vi "HCSD_125_scan.vi"() -> ()   [LabVIEW 2013]
uses:
  <vilib>/Utility/file.llb/Write To Spreadsheet File (string).vi
  <userlib>/caLab/Private/Get_PV-1D.vi
panel:
  in  "Diff SD":dbl=0.05
  out "refresh_ms":u32=51
  out "refresh (ms)":u32(graph)=51
  in  "diff HC":dbl=0.02 format="%#_13f"
  in  "stop":bool
  in  "Check period (ms)":u32=50 max=10
  out "Diff list":string[][](array[string])
  out "check loop":i32=1821
  out "EVENTs":i32
  out "Program Start Time":dbl=3594202634.3800077
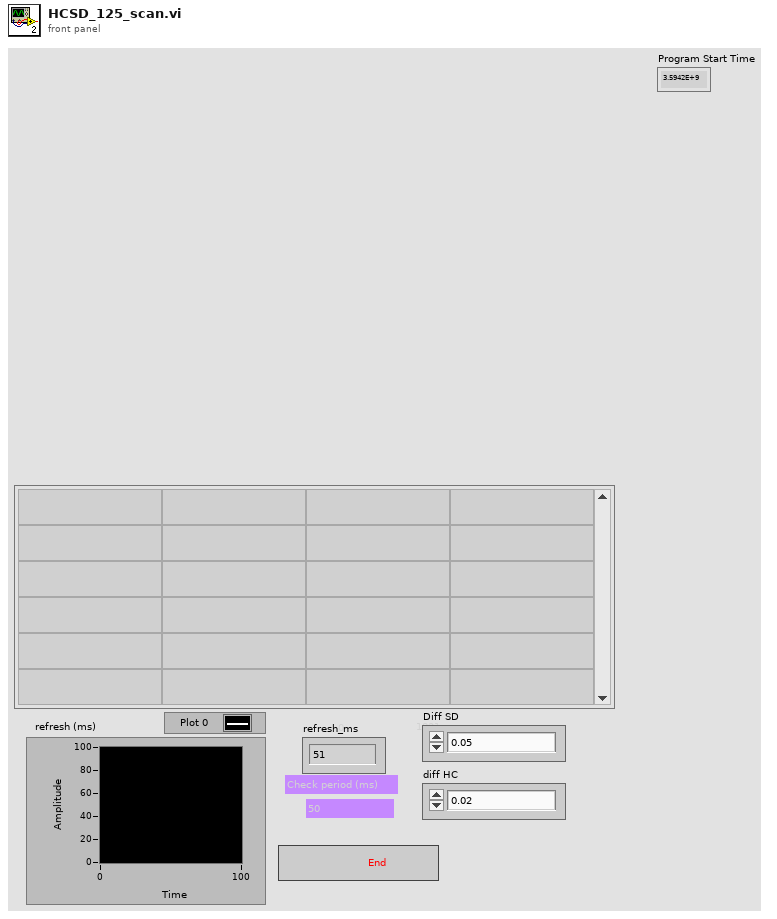
[diagram p1: front panel]
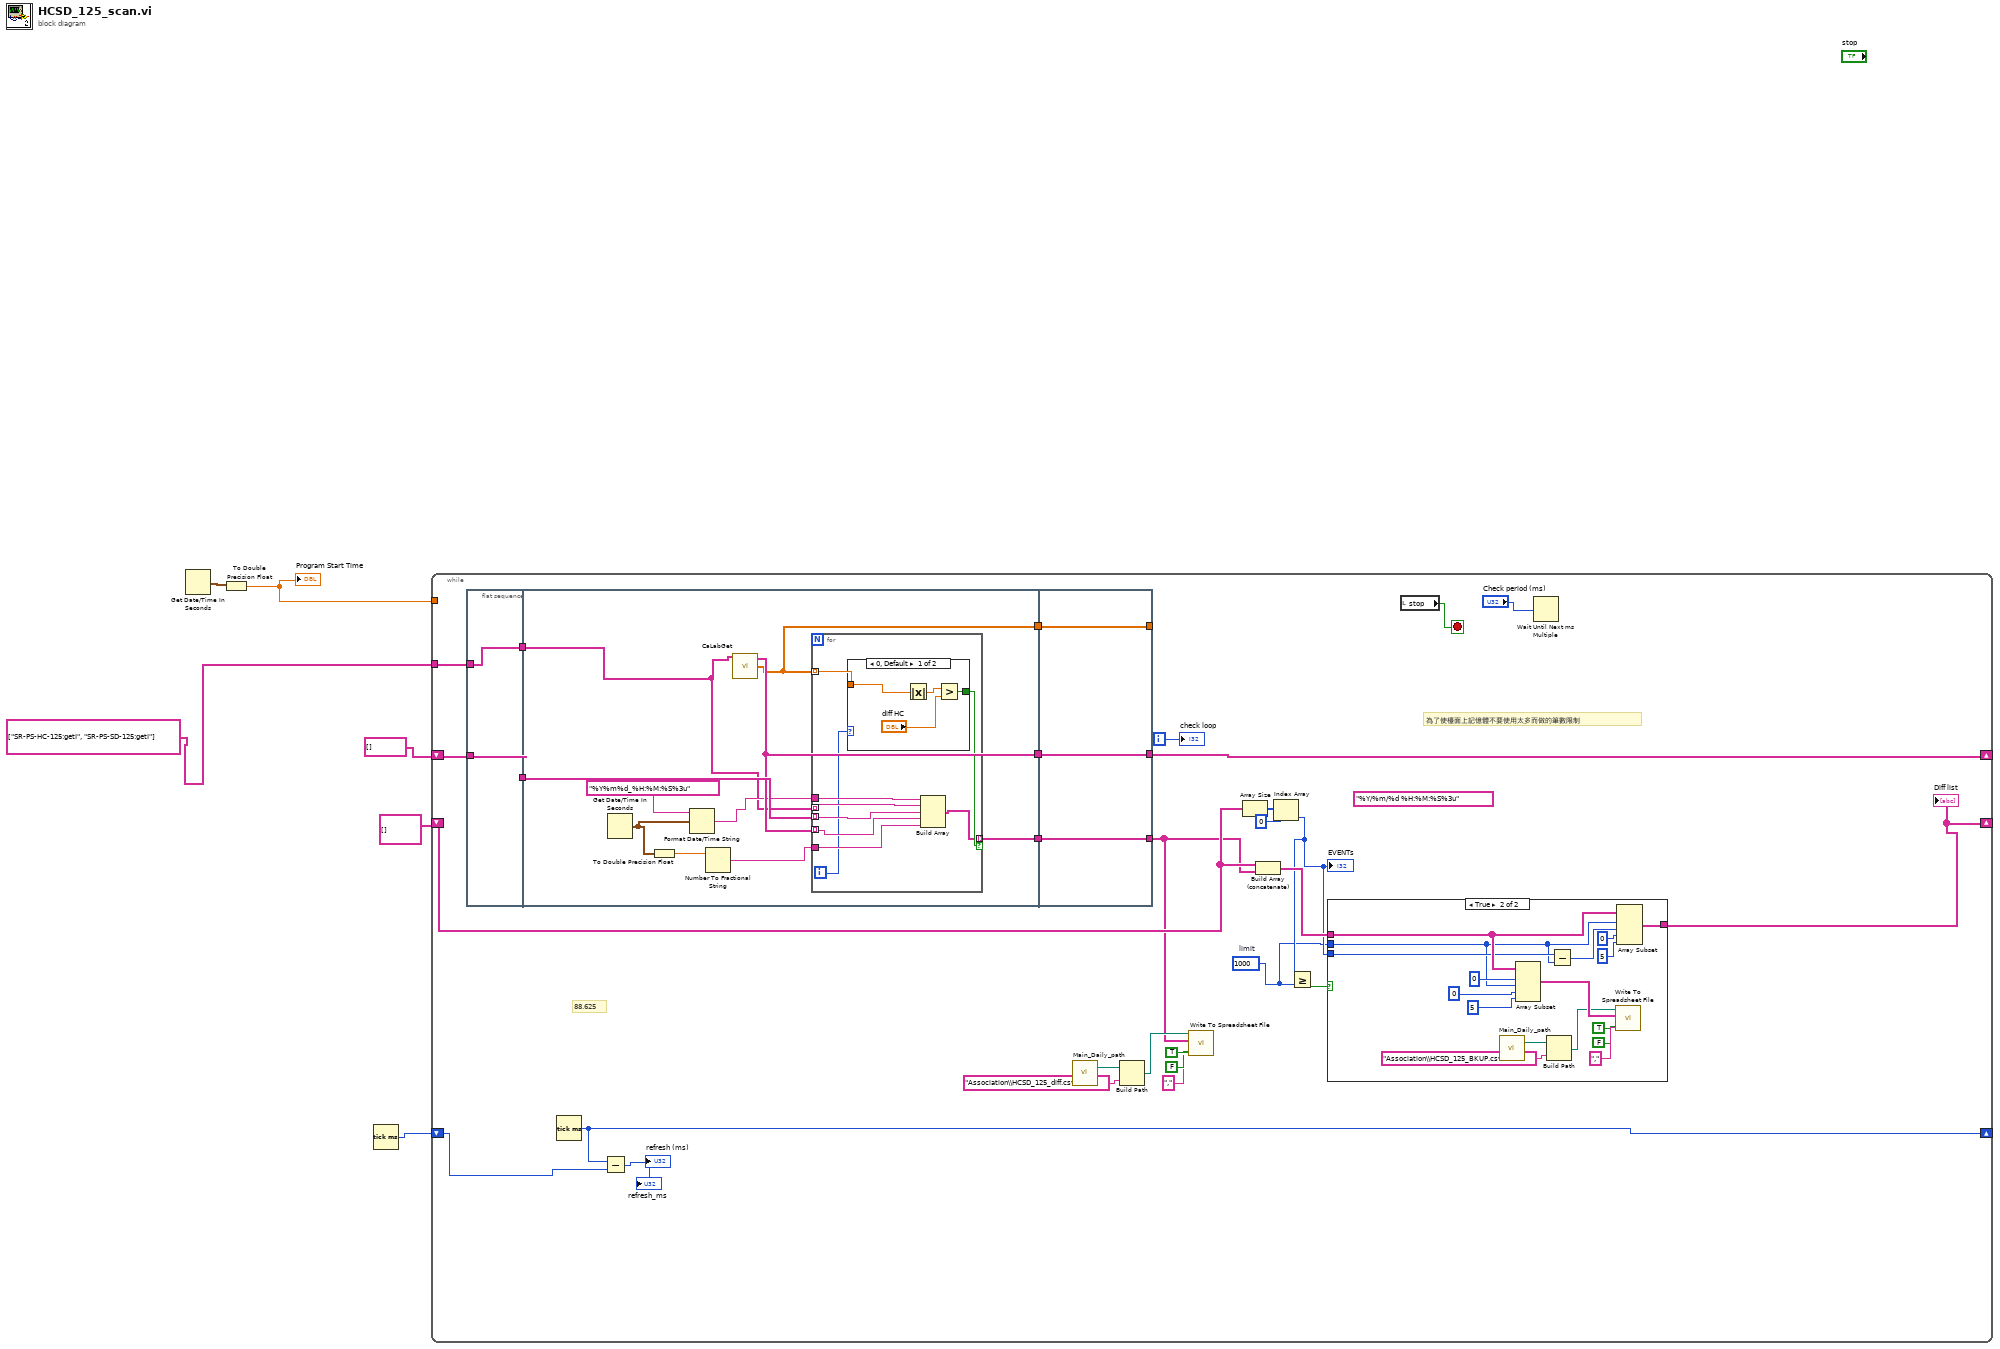
[diagram p0: block diagram]
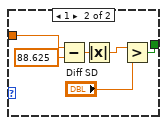
[diagram p3: hidden frame]
diagram:
  n1 = Get Date/Time In Seconds() -> (seconds since 1Jan1904=w5:timestamp)
  n2 = To Double Precision Float(number=w5) -> (double precision float=w6:dbl)
  "Program Start Time" <- w6
  n3 = Tick Count (ms)() -> (millisecond timer value=w1:u32)
  n4 = while {
    tunnel: w6 -> [_]
    shift-right: [w35] -> _
    shift-left: string[] [] -> [w32]
    shift-right: [w23] -> _
    shift-left: string[][] [] -> [w26]
    tunnel: string[] ["SR-PS-HC-125:getI", "SR-PS-SD-125:getI"] -> [w29]
    shift-right: [w15] -> _
    shift-left: w1 -> [w16]
    i -> [w27]
    stop <- w28 stop-if-true
    (unwired) "%Y/%m/%d %H:%M:%S%3u" ("time format string (%c)")
    w20 = 1000  # limit
    # "88.625"
    # "為了使檯面上記憶體不要使用太多而做的筆數限制"
    n5 = flat-sequence {
      tunnel: [w55] -> w33
      tunnel: w32 -> [w55]
      tunnel: [w54] -> w30
      tunnel: w29 -> [w54]
      tunnel: [w64] -> w34
      tunnel: w33 -> [w65]
      tunnel: [w58] -> w31
      tunnel: w30 -> [w57]
      tunnel: [w56] -> w17
      tunnel: [w87] -> w35
      tunnel: w34 -> [w87]
      tunnel: w31 -> [w86]
      tunnel: [w86] -> w7
      tunnel: [w85] -> _
      tunnel: w17 -> [w85]
      frame #0 {
      }
      frame #1 {
        n6 = Get Date/Time In Seconds() -> (seconds since 1Jan1904=w61:timestamp)
        n7 = To Double Precision Float(number=w61) -> (double precision float=w60:dbl)
        n8 = Format Date/Time String(time format string (%c)="%Y%m%d_%H:%M:%S%3u", seconds (now)=w61) -> (date/time string=w62:string)  [unwired: 1 in]
        n9 = Number To Fractional String(number=w60) -> (F-format string=w59:string)  [unwired: 3 in]
        n10 = call-poly <userlib>:"CaLabGet.vi"("PV Names"=w57) -> ("1rst Value (string)"=w64:string[], "1rst Value (number)"=w56:dbl[])  [unwired: 8 in, 5 out]
        n11 = for {
          tunnel: w65 -> [w71] mode=indexing
          tunnel: w64 -> [w70] mode=indexing
          tunnel: w57 -> [w74] mode=indexing
          tunnel: w62 -> [w73]
          tunnel: [w67] -> w58 mode=indexing if=w69
          tunnel: w59 -> [w72]
          tunnel: w56 -> [w68] mode=indexing
          i -> [w66]
          n12 = case shown="0, Default" w66 {
            tunnel: [w76 w80] -> w69
            tunnel: w68 -> [w75 w81]
            frame 0, Default {
              n13 = Absolute Value(x=w75) -> (abs(x)=w78:dbl)
              n14 = Greater?(x=w78, y="diff HC") -> (0:w76:bool)
            }
            frame 1 {
              n15 = Subtract(x=w81, y=88.625) -> (x-y=w84:dbl)
              n16 = Absolute Value(x=w84) -> (abs(x)=w83:dbl)
              n17 = Greater?(x=w83, y="Diff SD") -> (0:w80:bool)
            }
          }
          n18 = Build Array(w73, w74, w71, w70, w72) -> (w67:string[])
        }
      }
      frame #2 {
      }
    }
    n19 = Tick Count (ms)() -> (millisecond timer value=w15:u32)
    n20 = Subtract(x=w15, y=w16) -> (x-y=→"refresh (ms)" →"refresh_ms":u32)
    n21 = call "Main_Daily_path.vi"() -> ("Directory path"=w12:path)  [unwired: 10 in, 1 out]
    n22 = Build Path(base path=w12, name or relative path="Association\\HCSD_125_diff.csv" ("string")) -> (appended path=w13:path)
    n23 = call-poly <vilib>:"Write To Spreadsheet File.vi"("delimiter (\\t)"="," ("delimiter (\\t)"), "transpose? (no:F)"=FALSE, "append to file? (new file:F)"=TRUE, "2D data"=w7, "file path (dialog if empty)"=w13) -> ()  [unwired: 3 in, 1 out]
    n24 = Array Size(array=w26) -> (size(s)=w25:i32[])
    n25 = Build Array (concatenate)(w26, w7) -> (w22:string[][])
    n26 = Index Array(array=w25, index=0) -> (element=w21:i32)
    "EVENTs" <- w21
    n27 = Greater Or Equal?(x=w21, y=w20) -> (x >= y?=w19:bool)
    n28 = case shown="True" w19 {
      tunnel: w22 -> [w36 w47]
      tunnel: [w36 w51] -> w23
      tunnel: w21 -> [_ w42]
      tunnel: w20 -> [_ w41]
      frame False {
      }
      frame True {
        n29 = call "Main_Daily_path.vi"() -> ("Directory path"=w38:path)  [unwired: 10 in, 1 out]
        n30 = Array Subset(array=w47, index (row)=0 ("index"), length (row)=w41, index (col)=0 ("index"), length (col)=5 ("length")) -> (w46:string[][])
        n31 = Build Path(base path=w38, name or relative path="Association\\HCSD_125_BKUP.csv" ("string")) -> (appended path=w37:path)
        n32 = Subtract(x=w42, y=w41) -> (x-y=w40:i32)
        n33 = call-poly <vilib>:"Write To Spreadsheet File.vi"("delimiter (\\t)"="," ("delimiter (\\t)"), "transpose? (no:F)"=FALSE, "append to file? (new file:F)"=TRUE, "2D data"=w46, "file path (dialog if empty)"=w37) -> ()  [unwired: 3 in, 1 out]
        n34 = Array Subset(array=w47, index (row)=w41, length (row)=w40, index (col)=0 ("index"), length (col)=5 ("length")) -> (w51:string[][])
      }
    }
    "Diff list" <- w23
    n35 = local read "stop"() -> (w28:bool)
    n36 = Wait Until Next ms Multiple(millisecond multiple="Check period (ms)") -> ()  [unwired: 1 out]
    "check loop" <- w27
  }
